vi "get channels.vi"(11 "FPGA Module configuration in":refnum<class "FPGA Module configuration.lvclass">) -> (2 "channels":refnum<class "TBM channel.lvclass">[](array[class]), 3 "FPGA Module configuration out":refnum<class "FPGA Module configuration.lvclass">)   [LabVIEW 2014, in "FPGA Module configuration.lvclass"]
doc: "Returns an array of all Channels currently added to this configuration object."
uses:
  FPGA Module configuration.lvclass
  <vilib>/NI/Tag Bus Module Framework/channel/TBM channel.lvclass
  FPGA Module configuration.lvclass/FPGA Module configuration.ctl
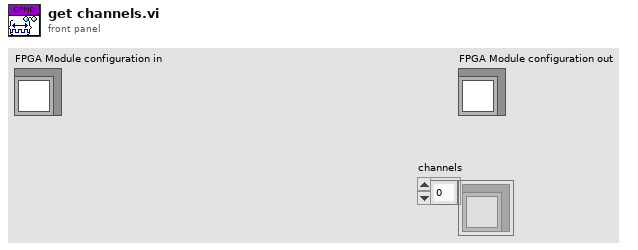
[diagram p1: front panel]
types:
  T1 = typedef "FPGA Module configuration.lvclass/Line.ctl" = cluster{"Channel":refnum<class "FPGA Channel.lvclass">}
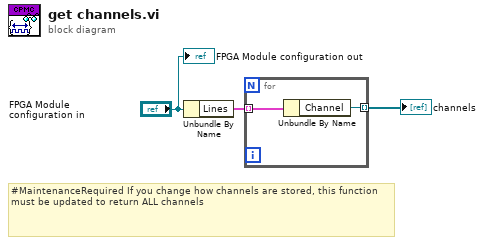
[diagram p0: block diagram]
diagram:
  # "#MaintenanceRequired If you change how channels are stored, this function must be updated to return ALL channels"
  n1 = Unbundle By Name("FPGA Module configuration in") -> ("Lines"=w2:T1[])
  n2 = for {
    tunnel: w2 -> [w5] mode=indexing
    tunnel: [w4] -> w1 mode=indexing
    n3 = Unbundle By Name(w5) -> ("Channel"=w4:refnum<class "FPGA Channel.lvclass">)
  }
  "channels" <- w1
  "FPGA Module configuration out" <- "FPGA Module configuration in"
